vi "Send Word Log Data.vi"(8 "error in (no error)":errorcluster, 10 "Data":T1[](array[typedef]), 11 "Producer in":refnum<class "Word Log Producer.lvclass">) -> (0 "error out":errorcluster, 3 "Producer out":refnum<class "Word Log Producer.lvclass">)   [LabVIEW 2020, in "Ballard ARINC 429 Engine.lvlib" / "Implementation.lvlib" / "Word Logging.lvlib"]
uses:
  Word Log Producer/Word Log Producer.lvclass
  Word.ctl
  Word Logging.lvlib
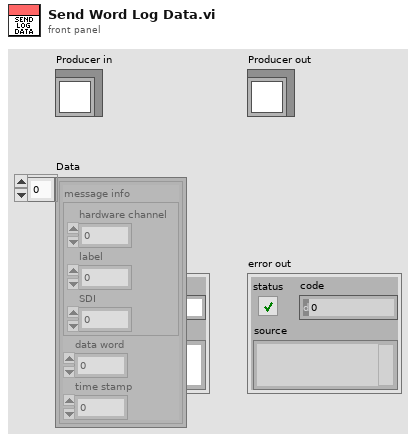
[diagram p1: front panel]
types:
  T1 = typedef "Ballard ARINC 429 Engine.lvlib/Implementation.lvlib/Word Logging.lvlib/Word.ctl" = cluster{"message info":cluster{"hardware channel":u8, "label":u8, "SDI":u8}, "data word":u32, "time stamp":dbl}
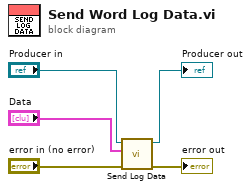
[diagram p0: block diagram]
diagram:
  n1 = call "Send Log Data.vi"("error in (no error)"="error in (no error)", "Data"="Data", "Word Log Producer in"="Producer in") -> ("error out"=→"error out":errorcluster, "Word Log Producer out"=→"Producer out":refnum<class "Word Log Producer.lvclass">)  [unwired: 7 in]
